vi "Get_Incorrectly_Classified_Imgs.vi"(6 "Dataset(In3D_Out1D)":T3, 7 "No_Of_Cols":i32, 8 "error in (no error)":errorcluster, 10 "Predictions":sgl[][](array[numeric]), 11 "MissClassed_idx":i32[](array[numeric])) -> (0 "error out":errorcluster, 3 "Images":T1[][](array[typedef]))   [LabVIEW 2020]
doc: "Helper VI for analysis.\nReturns Images as intensity graphs with the ground truth and corresponding predictions."
uses:
  Controls/Image_RGB.ctl
  <vilib>/Ngene/Deep Learning Toolkit/Toolkit/NN_Data/API/DataSet_Types/NN_DataSet(In3D_Out1D).ctl
  <vilib>/Ngene/Deep Learning Toolkit/Toolkit/NN_Data/API/DataRef_Types/NN_Data_ref(4D_SGL).ctl
  <vilib>/Ngene/Deep Learning Toolkit/Toolkit/NN_Data/API/DataRef_Types/NN_Data_ref(2D_SGL).ctl
  <vilib>/Ngene/Deep Learning Toolkit/Toolkit/NN_Data/API/DataRef_Types/NN_Data_ref(1D_I32).ctl
  <vilib>/Ngene/Deep Learning Toolkit/Toolkit/NN_Data/Controls/NN_Dims(C,H,W).ctl
  <vilib>/picture/picture.llb/Draw True-Color Pixmap.vi
  <vilib>/Ngene/Deep Learning Toolkit/Toolkit/Deep_Learning_Toolkit_by_Ngene.lvlib
panel:
  out "image":picture
  out "?":T1
  out "?":T2
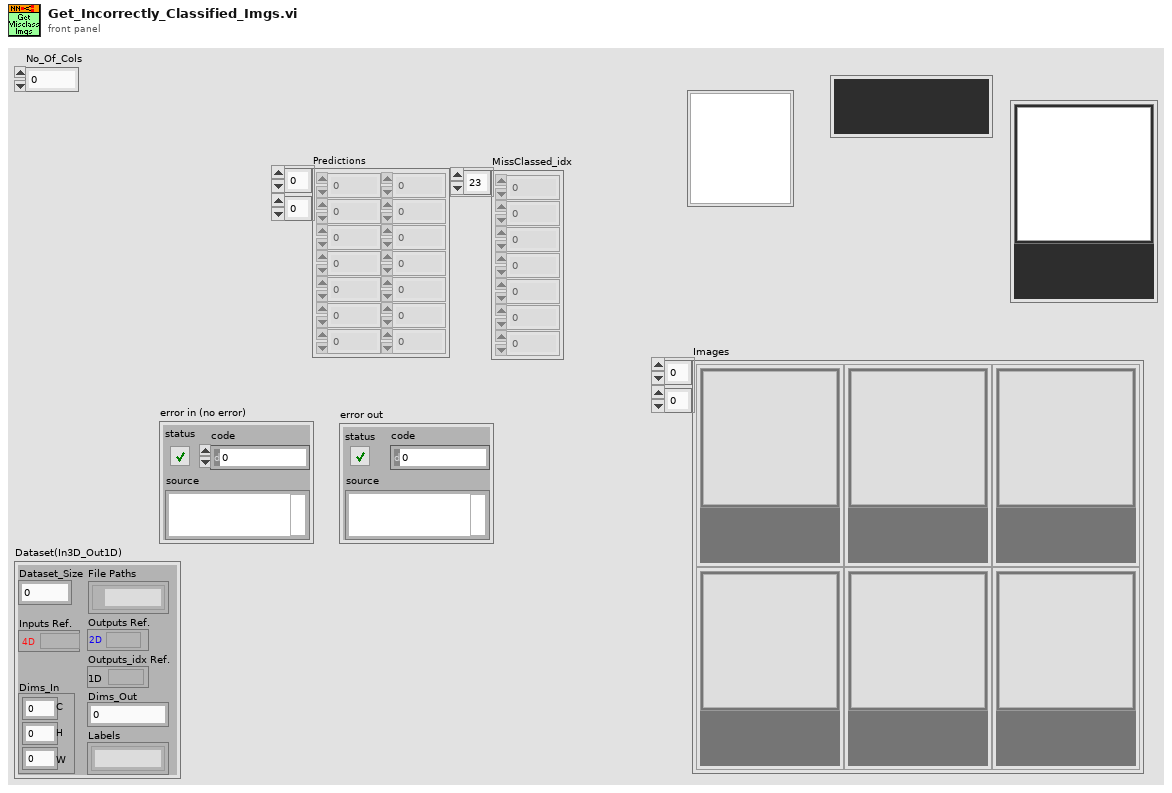
[diagram p1: front panel]
types:
  T1 = typedef "Image_RGB.ctl" = cluster{"image":picture, "Truth":string, "Predicted":string, "Filename":string}
  T2 = cluster{"Truth":string, "Predicted":string, "Filename":string}
  T3 = typedef "Deep_Learning_Toolkit_by_Ngene.lvlib/NN_DataSet(In3D_Out1D).ctl" = cluster{"Inputs Ref.":T4, "Outputs Ref.":T5, "Dataset_Size":i32, "Outputs_idx Ref.":T6, "Dims_In":T7, "Dims_Out":i32, "Labels":string[], "File Paths":path[]}
  T4 = typedef "Deep_Learning_Toolkit_by_Ngene.lvlib/NN_Data_ref(4D_SGL).ctl" = refnum<data-value>
  T5 = typedef "Deep_Learning_Toolkit_by_Ngene.lvlib/NN_Data_ref(2D_SGL).ctl" = refnum<data-value>
  T6 = typedef "Deep_Learning_Toolkit_by_Ngene.lvlib/NN_Data_ref(1D_I32).ctl" = refnum<data-value>
  T7 = typedef "Deep_Learning_Toolkit_by_Ngene.lvlib/NN_Dims(C,H,W).ctl" = cluster{"C":i32, "H":i32, "W":i32}
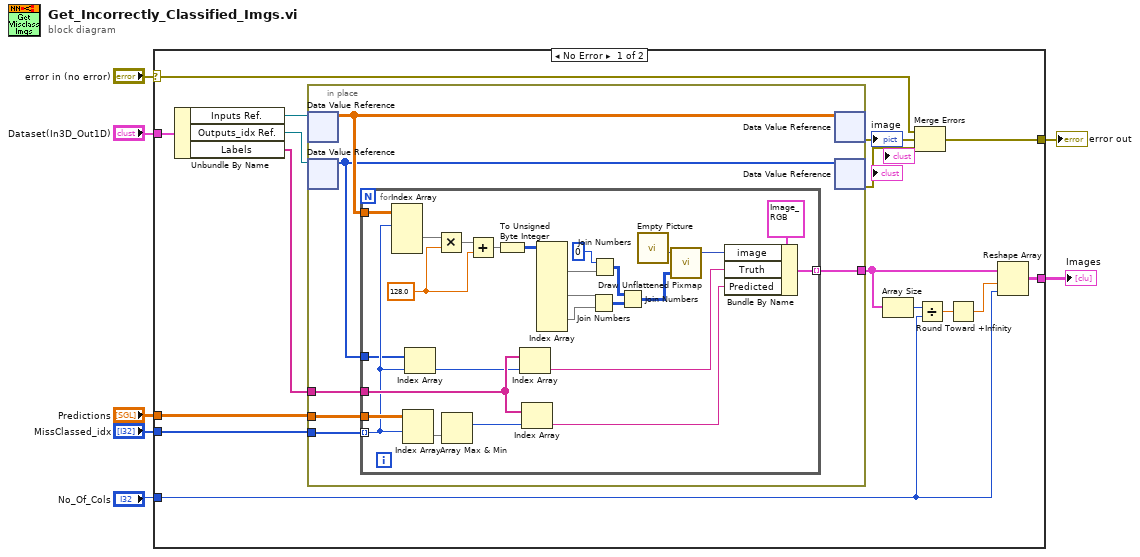
[diagram p0: block diagram]
diagram:
  n1 = case shown="No Error" "error in (no error)" {
    selector: "error in (no error)" -> [w19 w56]
    tunnel: [w18 w56] -> w7
    tunnel: "Dataset(In3D_Out1D)" -> [w13 _]
    tunnel: "Predictions" -> [w12 _]
    tunnel: "MissClassed_idx" -> [w11 _]
    tunnel: [w10 _] -> w2
    tunnel: "No_Of_Cols" -> [w9 _]
    frame No Error {
      n2 = Unbundle By Name(w13) -> ("Inputs Ref."=w22:T4, "Outputs_idx Ref."=w21:T6, "Labels"=w8:string[])
      n3 = in-place {
        in-place-border: w11 -> [w25]
        in-place-border: w12 -> [w27]
        in-place-border: w8 -> [w26]
        in-place-border: [w24] -> w14
        n4 = in-place-dvr #1(w22) -> (w29:sgl[][][][])  [unwired: 1 out]
        n5 = in-place-dvr #2(w21) -> (w28:i32[])  [unwired: 1 out]
        n6 = for {
          tunnel: w29 -> [w55]
          tunnel: w25 -> [w39] mode=indexing
          tunnel: w28 -> [w36]
          tunnel: w27 -> [w54]
          tunnel: w26 -> [w52]
          tunnel: [w46] -> w24 mode=indexing
          w31 = sgl 128.0 ("x")
          n7 = Index Array(array=w55, index (dim 0)=w39) -> (element=w34:sgl[][][])  [unwired: 3 in]
          n8 = Index Array(array=w54, index (row)=w39) -> (element=w53:sgl[])  [unwired: 1 in]
          n9 = Index Array(array=w36, index=w39) -> (element=w35:i32)
          n10 = Multiply(x=w34, y=w31) -> (x*y=w33:sgl[][][])
          n11 = Array Max & Min(array=w53) -> (max index (indices)=w37:i32)  [unwired: 3 out]
          n12 = Add(x=w33, y=w31) -> (x+y=w32:sgl[][][])
          n13 = To Unsigned Byte Integer(number=w32) -> (unsigned 8bit integer=w30:u8[][][])
          n14 = Index Array(array=w52, index=w35) -> (element=w38:string)
          n15 = Index Array(array=w52, index=w37) -> (element=w40:string)
          n16 = Index Array(array=w30) -> (element #1=w43:u8[][], element #2=w41:u8[][], element #3=w42:u8[][])  [unwired: 9 in]
          n17 = Join Numbers(hi=w41, lo=w42) -> ((hi.lo)=w49:u16[][])
          n18 = Join Numbers(hi=u8 0 ("element"), lo=w43) -> ((hi.lo)=w50:u16[][])
          n19 = Join Numbers(hi=w50, lo=w49) -> ((hi.lo)=w44:u32[][])
          n20 = call "Empty Picture"() -> ("empty picture"=w51:picture)
          n21 = call-poly <vilib>:"Draw Unflattened Pixmap.vi"("picture"=w51, "data (RGB format)"=w44) -> ("new picture"=w47:picture)  [unwired: 7 in]
          n22 = Bundle By Name(cluster=T1 {"image"=bytes[0], "Truth"="", "Predicted"="", "Filename"=""}, "image"=w47, "Truth"=w38, "Predicted"=w40) -> (w46:T1)
        }
        n23 = in-place-dvr #1(w29) -> (w23:errorcluster)  [unwired: 1 out]
        n24 = in-place-dvr #2(w28) -> (w20:errorcluster)  [unwired: 1 out]
      }
      n25 = Array Size(array=w14) -> (size(s)=w16:i32)
      n26 = Merge Errors(w19, w23, w20) -> (w18:errorcluster)
      n27 = Divide(x=w16, y=w9) -> (x/y=w17:dbl)
      n28 = Round Toward +Infinity(x=w17) -> (ceil(x): smallest int >= x=w15:dbl)
      n29 = Reshape Array(w14, w15, w9) -> (w10:T1[][])
    }
    frame Error {
    }
  }
  "error out" <- w7
  "Images" <- w2
